vi "Read Drag Mode.vi"(8 "error in (no error)":errorcluster, 11 "ControlDragStartingMsg In":refnum<class "ControlDragStartingMsg.lvclass">) -> (0 "error out":errorcluster, 2 "Drag Mode":enum32{"copy or move", "copy only", "move only"}(ring), 3 "ControlDragStartingMsg Out":refnum<class "ControlDragStartingMsg.lvclass">)   [LabVIEW 2017, in "ActorEvents.lvlib" / "ControlDragStartingMsg.lvclass"]
uses:
  <vilib>/gpm_packages/@cs/mva-viewable/Source/ActorEvents/IEventAggregator Messages/ControlDragStartingMsg/ControlDragStartingMsg.lvclass
  <vilib>/gpm_packages/@cs/mva-viewable/Source/ActorEvents/IEventAggregator Messages/ControlDragStartingMsg/ControlDragStartingMsg.lvclass/ControlDragStartingMsg.ctl
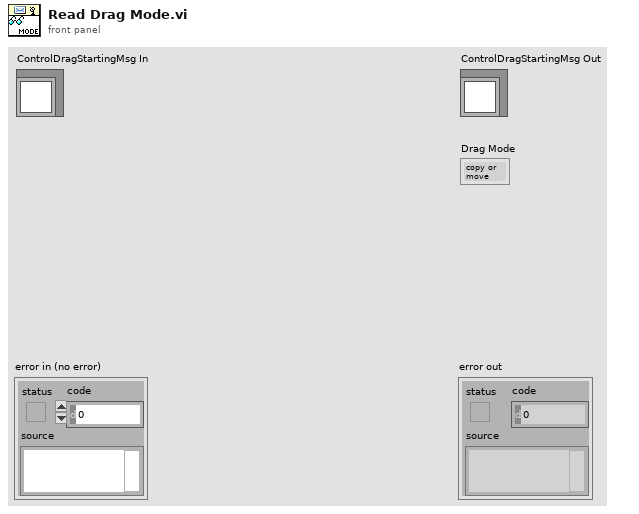
[diagram p1: front panel]
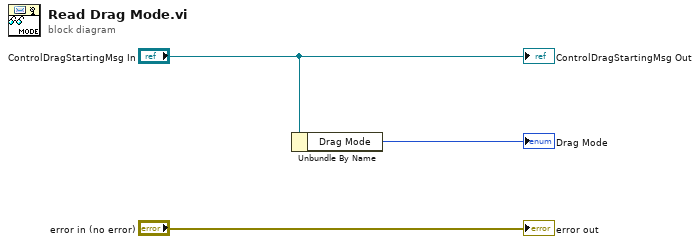
[diagram p0: block diagram]
diagram:
  n1 = Unbundle By Name("ControlDragStartingMsg In") -> ("Drag Mode"=→"Drag Mode":enum32{"copy or move", "copy only", "move only"})
  "error out" <- "error in (no error)"
  "ControlDragStartingMsg Out" <- "ControlDragStartingMsg In"
